vi "poly_lock_fp_updates_lock_self.vi"(8 "error in":errorcluster) -> (0 "error out":errorcluster)   [LabVIEW 2015]
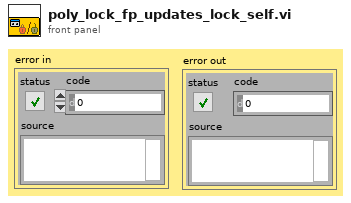
[diagram p1: front panel]
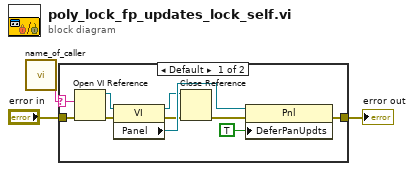
[diagram p0: block diagram]
diagram:
  n1 = call "name_of_caller.vi"() -> ("name of caller out"=w1:string)  [unwired: 4 in]
  n2 = case shown="Default" w1 {
    selector: w1 -> [w10 _]
    tunnel: [w12 w14] -> w3
    tunnel: "error in" -> [w8 w14]
    frame Default {
      n3 = Open VI Reference(vi path=w10, error in (no error)=w8) -> (vi reference=w9:refnum<vi>, error out=w7:errorcluster)  [unwired: 4 in]
      n4 = property class="VI"(reference=w9, error in=w7) -> (reference out=w6:refnum<vi>, error out=w5:errorcluster, "Panel"=w11:refnum<vi>)
      n5 = Close Reference(reference=w6, error in (no error)=w5) -> (error out=w4:errorcluster)
      n6 = property class="Pnl"(reference=w11, error in=w4, "DeferPanUpdts"=TRUE) -> (error out=w12:errorcluster)  [unwired: 1 out]
    }
    frame "" {
    }
  }
  "error out" <- w3
